vi "阀配置写入.vi"(8 "error in (no error)":errorcluster caption="错误输入（无错误）", 10 "data":T1 {"Value" items=["三通阀", "排阀"]}, 11 "SingleStepTestV3 输入":refnum<class "SingleStepCODMnV2.lvclass">) -> (0 "error out":errorcluster caption="错误输出", 3 "SingleStepTestV3 输出":refnum<class "SingleStepCODMnV2.lvclass">)   [LabVIEW 2016, in "SingleStepCODMnV2.lvlib" / "SingleStepCODMnV2.lvclass"]
uses:
  SingleStepCODMnV2.lvclass
  SingleStepCODMnV2.lvclass/SingleStepCODMnV2.ctl
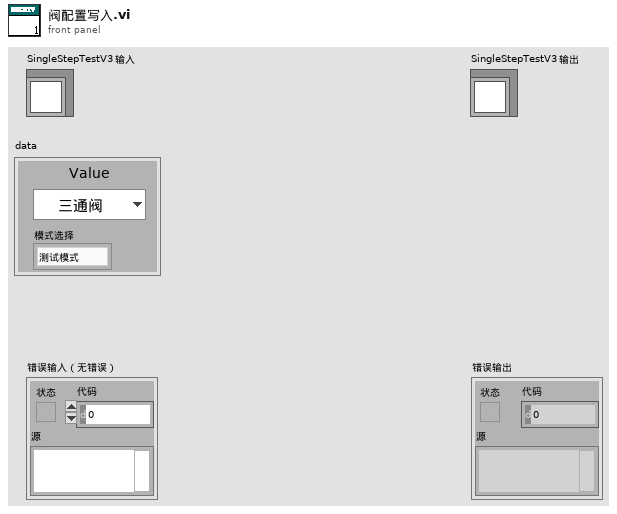
[diagram p1: front panel]
types:
  T1 = cluster{"Value":u8, "模式选择":enum16{"测试模式", "流程模式"}}
  T2 = enum8{"Enabled", "Disabled", "Disabled and Grayed Out"}
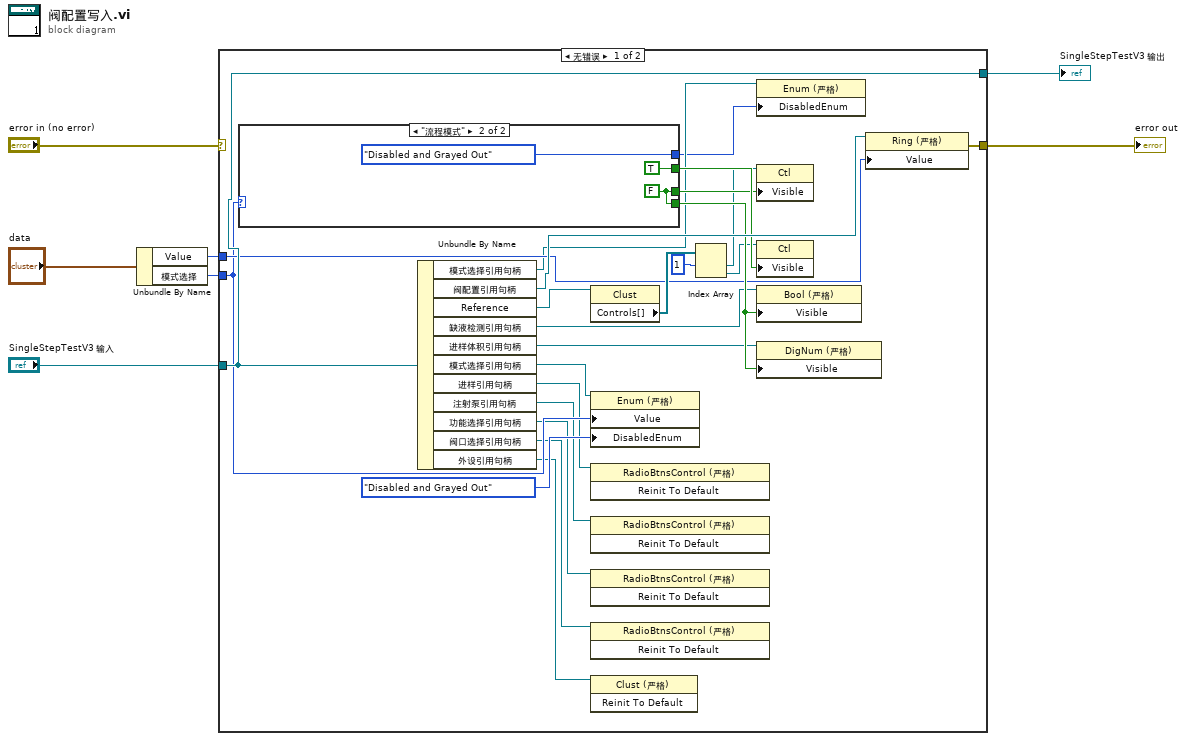
[diagram p0: block diagram]
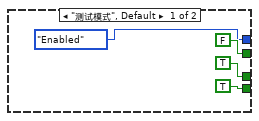
[diagram p2: hidden frame]
diagram:
  n1 = Unbundle By Name("data") -> ("Value"=w2:u8, "模式选择"=w1:enum16{"测试模式", "流程模式"})
  n2 = case shown="无错误" "error in (no error)" {
    selector: "error in (no error)" -> [_ w40]
    tunnel: [w29 w40] -> w6
    tunnel: [w30 w39] -> w4
    tunnel: "SingleStepTestV3 输入" -> [w30 w39]
    tunnel: w2 -> [w16 _]
    tunnel: w1 -> [w15 _]
    frame No Error {
      n3 = case shown="\"流程模式\"" w15 {
        tunnel: [TRUE w37] -> w26
        tunnel: [FALSE TRUE] -> w27
        tunnel: [TRUE ("可见") w37] -> w28
        tunnel: [T2."Enabled" ("禁用") T2."Disabled and Grayed Out" ("禁用")] -> w13
        frame "测试模式", Default {
        }
        frame "流程模式" {
          w37 = FALSE
        }
      }
      n4 = Unbundle By Name(w30) -> ("模式选择引用句柄"=w14:refnum<vi>, "阀配置引用句柄"=w31:refnum<vi>, "Reference"=w21:refnum<vi>, "缺液检测引用句柄"=w20:refnum<vi>, "进样体积引用句柄"=w19:refnum<vi>, "模式选择引用句柄"=w18:refnum<vi>, "进样引用句柄"=w12:refnum<vi>, "注射泵引用句柄"=w11:refnum<vi>, "功能选择引用句柄"=w10:refnum<vi>, "阀口选择引用句柄"=w9:refnum<vi>, "外设引用句柄"=w8:refnum<vi>)
      n5 = property class="Clust"(reference=w21) -> ("Controls[]"=w23:refnum<vi>[])  [unwired: 1 in, 2 out]
      n6 = property class="Enum (严格)"(reference=w18, "Value"=w15, "DisabledEnum"=T2."Disabled and Grayed Out" ("禁用")) -> ()  [unwired: 1 in, 2 out]
      n7 = invoke class="RadioBtnsControl (严格)" method="Reinit To Default"(reference=w12) -> ()  [unwired: 2 in, 3 out]
      n8 = invoke class="RadioBtnsControl (严格)" method="Reinit To Default"(reference=w11) -> ()  [unwired: 2 in, 3 out]
      n9 = invoke class="RadioBtnsControl (严格)" method="Reinit To Default"(reference=w10) -> ()  [unwired: 2 in, 3 out]
      n10 = invoke class="RadioBtnsControl (严格)" method="Reinit To Default"(reference=w9) -> ()  [unwired: 2 in, 3 out]
      n11 = invoke class="Clust (严格)" method="Reinit To Default"(reference=w8) -> ()  [unwired: 2 in, 3 out]
      n12 = Index Array(array=w23, index #1=1 ("索引")) -> (element #1=w24:refnum<vi>, element #2=w25:refnum<vi>)  [unwired: 1 in]
      n13 = property class="Enum (严格)"(reference=w14, "DisabledEnum"=w13) -> ()  [unwired: 1 in, 2 out]
      n14 = property class="Ctl"(reference=w24, "Visible"=w26) -> ()  [unwired: 1 in, 2 out]
      n15 = property class="Ctl"(reference=w25, "Visible"=w27) -> ()  [unwired: 1 in, 2 out]
      n16 = property class="Bool (严格)"(reference=w20, "Visible"=w28) -> ()  [unwired: 1 in, 2 out]
      n17 = property class="DigNum (严格)"(reference=w19, "Visible"=w28) -> ()  [unwired: 1 in, 2 out]
      n18 = property class="Ring (严格)"(reference=w31, "Value"=w16) -> (error out=w29:errorcluster)  [unwired: 1 in, 1 out]
    }
    frame Error {
    }
  }
  "error out" <- w6
  "SingleStepTestV3 输出" <- w4
